vi "Get or Add Workbook.vi"(8 "error in":errorcluster, 11 "Workbookpart in":refnum<k24>) -> (0 "error out":errorcluster, 2 "Workbook":refnum<k24>, 3 "Workbookpart out":refnum<k24>)   [LabVIEW 2021, in "Open Xml.lvlib"]
uses:
  Open Xml.lvlib
  D:/git/Open-Xml-LabVIEW/dll/DocumentFormat.OpenXml.dll
  dll/DocumentFormat.OpenXml.dll
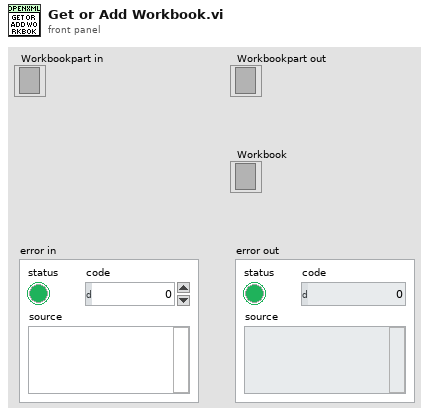
[diagram p1: front panel]
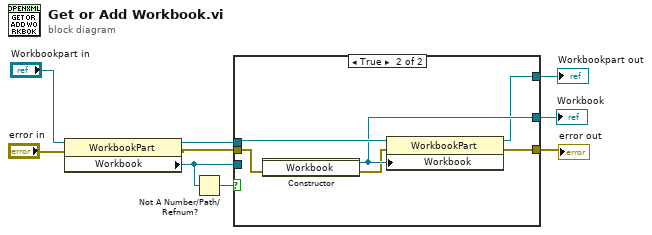
[diagram p0: block diagram]
diagram:
  n1 = property class="WorkbookPart"(reference="Workbookpart in", error in="error in") -> (reference out=w2:refnum<k24>, error out=w6:errorcluster, "Workbook"=w5:refnum<k24>)
  n2 = Not A Number/Path/Refnum?(number/path/refnum=w5) -> (NaN/Path/Refnum?=w7:bool)
  n3 = case shown="True" w7 {
    tunnel: w6 -> [w12 w15]
    tunnel: w5 -> [w10 _]
    tunnel: [w10 w16] -> w3
    tunnel: [w12 w18] -> w4
    tunnel: w2 -> [w11 w17]
    tunnel: [w11 w13] -> w1
    frame False {
    }
    frame True {
      n4 = constructor class="Workbook"(error in=w15) -> (reference out=w16:refnum<k24>, error out=w14:errorcluster)  [unwired: 2 in, 1 out]
      n5 = property class="WorkbookPart"(reference=w17, error in=w14, "Workbook"=w16) -> (reference out=w13:refnum<k24>, error out=w18:errorcluster)
    }
  }
  "error out" <- w4
  "Workbook" <- w3
  "Workbookpart out" <- w1
